vi "Do.vi"(8 "error in":errorcluster, 10 "Actor in":refnum<class "Actor.lvclass">, 11 "Change Inlet MSG":refnum<class "Change Inlet MSG.lvclass">) -> (0 "error out":errorcluster, 2 "Actor out":refnum<class "Actor.lvclass">)   [LabVIEW 2014, in "Controller.lvlib" / "Change Inlet MSG.lvclass"]
doc: "(<B>Filename</B>: Actor Framework.lvlib:Message.lvclass:Do.vi)\n\nDefines what a message does when it is received by an actor. Generally, a message instructs an actor to invoke one of its methods. By default, this method does nothing. A child class must override it to define behavior. Create a child class by using the Actor Framework Message Maker dialog box."
uses:
  Change Inlet MSG.lvclass
  <vilib>/ActorFramework/Actor/Actor.lvclass
  Controller.lvclass
  Update Switch State MSG/Update Switch MSG.lvclass/Update Switch MSG.ctl
  SuperActor/SuperActor.lvclass/SuperActor.ctl
  Update Switch State MSG/Read SwitchState.vi
  SuperActor/Read CVT Session.vi
  SuperActor/Read Log Session.vi
  <vilib>/DAQmx/write.llb/DAQmx Write (Digital 1D Bool NChan 1Samp 1Line).vi
  <vilib>/DAQmx/write.llb/DAQmx Write (Digital Bool 1Line 1Point).vi
  <userlib>/_Session Fwk/Session - Root.lvclass
  reusable/Session APIs/Session Log/System Log.lvclass
  reusable/Session APIs/CVT/CVT.lvclass
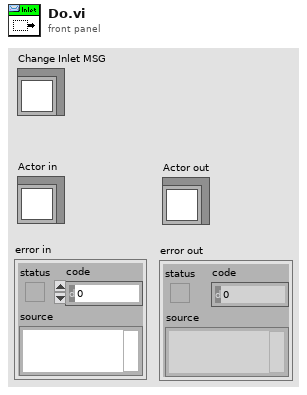
[diagram p1: front panel]
types:
  T1 = typedef "Session - Root.lvclass/Session Handle.ctl" = refnum<data-value>
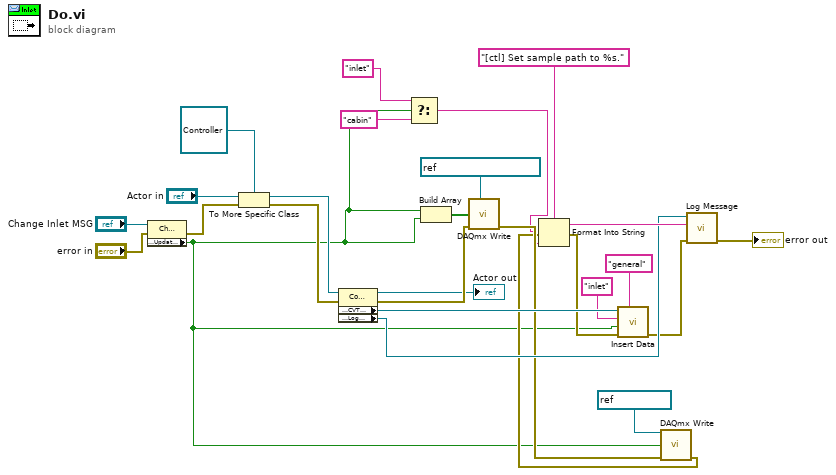
[diagram p0: block diagram]
diagram:
  n1 = property class="Change Inlet MSG.lvclass"(reference="Change Inlet MSG", error in="error in") -> (error out=w18:errorcluster, "Accessors:UpdateSw"=w4:bool)  [unwired: 1 out]
  n2 = To More Specific Class(target class=refnum<class "Controller.lvclass"> refnum ("Controller.lvlib:Controller"), reference="Actor in", error in=w18) -> (specific class reference=w17:refnum<class "Controller.lvclass">, error out=w11:errorcluster)
  n3 = property class="Controller"(reference=w17, error in=w11) -> (reference out=→"Actor out":refnum<class "Controller.lvclass">, error out=w16:errorcluster, "Accessors:CVT Session"=w14:T1, "Accessors:Log Session"=w10:T1)
  n4 = Select(t="inlet", s=w4, f="cabin") -> (s? t:f=w1:string)
  n5 = Build Array(w4, w4) -> (w27:bool[])
  n6 = call-poly <vilib>:"DAQmx Write.vi"("task/channels in"=refnum<k21> "Cabin Valve CMD", "data"=w27, "error in"=w16) -> ("error out"=w6:errorcluster)  [unwired: 10 in, 2 out]
  n7 = call-poly <vilib>:"DAQmx Write.vi"("task/channels in"=refnum<k21> "Inlet LED", "data"=w4, "error in"=w6) -> ("error out"=w5:errorcluster)  [unwired: 10 in, 2 out]
  n8 = Format Into String(format string="[ctl] Set sample path to %s.", error in=w5, w1) -> (resulting string=w22:string, error out=w9:errorcluster)  [unwired: 1 in]
  n9 = call "Insert Data.vi"("Group"="general", "error in"=w9, "Data"=w4, "tag"="inlet", "CVT Session In"=w14) -> ("error out"=w8:errorcluster)  [unwired: 5 in, 1 out]
  n10 = call "Log Message.vi"("error in"=w8, "MSG In"=w22, "session in"=w10) -> ("error out"=→"error out":errorcluster)  [unwired: 7 in, 1 out]
